vi "Pause.vi"(8 "error in":errorcluster, 11 "Tacmina Settings in":T1) -> (0 "error out":errorcluster, 3 "Tacmina Settings out":T1)   [LabVIEW 2018, in "Tacmina QI.lvlib"]
uses:
  Tacmina QI.lvlib
  Tacmina QI DAQ Setting.ctl
  <vilib>/DAQmx/write.llb/DAQmx Write (Digital Bool 1Line 1Point).vi
  <vilib>/DAQmx/write.llb/DAQmx Write (Analog DBL 1Chan 1Samp).vi
  <vilib>/DAQmx/miscellaneous.llb/DAQmx Fill In Error Info.vi
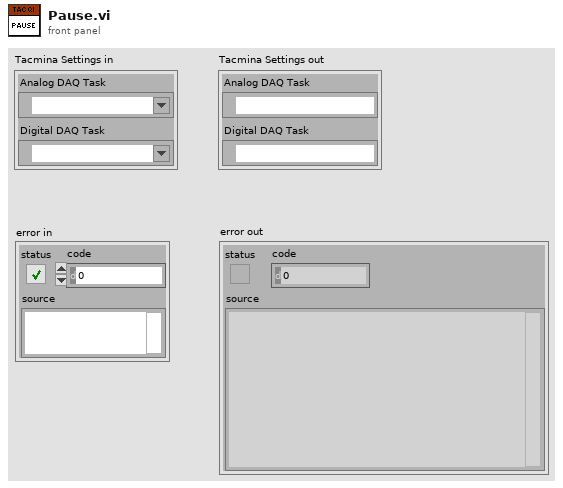
[diagram p1: front panel]
types:
  T1 = typedef "Tacmina QI.lvlib/Tacmina QI DAQ Setting.ctl" = cluster{"Analog DAQ Task":refnum<k21>, "Digital DAQ Task":refnum<k21>}
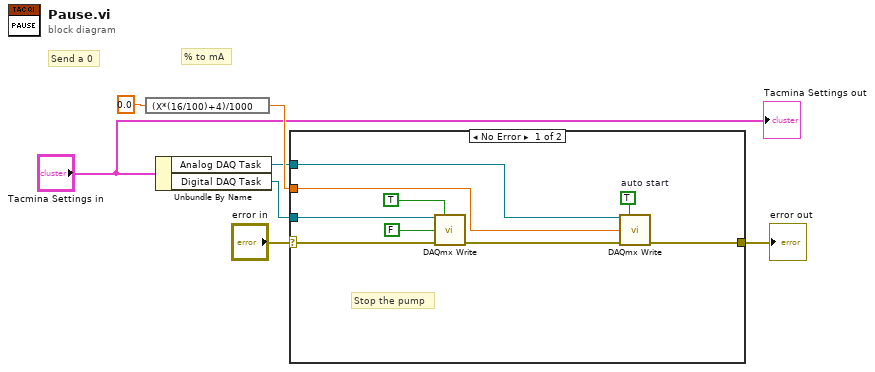
[diagram p0: block diagram]
diagram:
  # "Send a 0"
  # "% to mA"
  n1 = expression code="(X*(16/100)+4)/1000"(0.0 ("speed")) -> (w7:dbl)
  n2 = Unbundle By Name("Tacmina Settings in") -> ("Analog DAQ Task"=w4:refnum<k21>, "Digital DAQ Task"=w5:refnum<k21>)
  n3 = case shown="No Error" "error in" {
    selector: "error in" -> [w8 w17]
    tunnel: w5 -> [w16 _]
    tunnel: w7 -> [w9 _]
    tunnel: w4 -> [w15 _]
    tunnel: [w10 w17] -> w2
    frame No Error {
      w13 = TRUE  # auto start
      # "Stop the pump"
      n4 = call-poly <vilib>:"DAQmx Write.vi"("task/channels in"=w16, "auto start"=TRUE, "data"=FALSE, "error in"=w8) -> ("error out"=w11:errorcluster)  [unwired: 9 in, 2 out]
      n5 = call-poly <vilib>:"DAQmx Write.vi"("task/channels in"=w15, "auto start"=w13, "data"=w9, "error in"=w11) -> ("error out"=w10:errorcluster)  [unwired: 9 in, 2 out]
    }
    frame Error {
    }
  }
  "error out" <- w2
  "Tacmina Settings out" <- "Tacmina Settings in"
